vi "Ec. estados.vi"() -> ()   [LabVIEW 2020]
uses:
  <vilib>/addons/Control Design/_Model Construction/Data Typedefs.llb/CD Time Info.ctl
  <vilib>/addons/Control Design/_Model Construction/Model Creation.llb/Model Creation SubVI/cd_Create State Space Model.vi
  <vilib>/addons/Control Design/_Model Construction/Model Creation.llb/Model Creation SubVI/cd_Create Transfer Function Model.vi
  <vilib>/addons/Control Design/_Model Conversions/Model Type.llb/Model Conversion SubVI/cd_Convert Transfer Function to State-Space Model.vi
  <vilib>/addons/Control Design/_Utility/Model Viewer.llb/Model Viewer SubVI/cd_Draw State-Space Equation (SS).vi
  <vilib>/addons/Control Design/_Dynamic Analysis/Dynamic Analysis.llb/Dynamic Analysis subVI/cd_Poles (State-Space).vi
  <vilib>/addons/Control Design/_Utility/Model Viewer.llb/Model Viewer SubVI/cd_Draw Transfer Function Equation (SS).vi
  <vilib>/imath/engines/lvmath2/RunTimeEngine/Managers/WorkSpace/UID Generator.vi
  <vilib>/imath/engines/lvmath/Plug In/Control Design/BuiltInFunctions/ackermann/NIMS_CD_ackermann(A,B,poles,STR).vi
  <vilib>/imath/engines/lvmath2/RunTimeEngine/RunTimeType/NIMS_RunTimeType_From StrictType (excl LVString).vi
  <instcachedir>/0/NIMS_RunTimeType_From StrictType (excl LVString)_283B1B2000484AAA8744D21CE97EA49F.lvgen/NIMS_RunTimeType_From StrictType (excl LVString)_283B1B2000484AAA8744D21CE97EA49F_000.vi
  <vilib>/imath/engines/lvmath2/RunTimeEngine/LocalVariableDefStatement/MC_LocalVariableDefStatement_Display.vi
  <vilib>/imath/engines/lvmath2/RunTimeEngine/ArithmeticOperatorToken/NIMS_ArithmeticOperator_multmx.vi
  <instcachedir>/0/NIMS_ArithmeticOperator_multmx_177F0753FB7A49B190E35F5DD0E80316.lvgen/NIMS_ArithmeticOperator_multmx_177F0753FB7A49B190E35F5DD0E80316_004.vi
  <vilib>/imath/engines/lvmath2/RunTimeEngine/ArithmeticOperatorToken/NIMS_ArithmeticOperator_minus.vi
  <instcachedir>/0/NIMS_ArithmeticOperator_minus_822089A08BE049DB927E6BEA78E100F1.lvgen/NIMS_ArithmeticOperator_minus_822089A08BE049DB927E6BEA78E100F1_002.vi
  <vilib>/imath/engines/lvmath2/RunTimeSupport/NIMS_Get Scalar_w Error.vi
  <instcachedir>/0/NIMS_Get Scalar_w Error_5A0E401CB6154DCF81784DB8E431B6E1.lvgen/NIMS_Get Scalar_w Error_5A0E401CB6154DCF81784DB8E431B6E1_003.vi
  <vilib>/imath/engines/lvmath2/RunTimeEngine/BuiltInFunctions/ss_to_tf/NIMS_ss_to_tf(4i).vi
  <vilib>/imath/engines/lvmath2/RunTimeEngine/ErrorHandling/NIMS_Create Error From Enums.vi
  <vilib>/imath/engines/lvmath/Plug In/Control Design/BuiltInFunctions/tf/NIMS_CD_tf(num,den,Ts).vi
  <vilib>/imath/engines/lvmath/Plug In/Control Design/BuiltInFunctions/tf/NIMS_CD_tf(K,Ts).vi
  <vilib>/imath/engines/lvmath2/RunTimeEngine/VariableToken/NIMS_VariableToken_CondDefined.vi
  <instcachedir>/0/NIMS_VariableToken_CondDefined_537E119D71C74F9D9452D6FF923F1E1F.lvgen/NIMS_VariableToken_CondDefined_537E119D71C74F9D9452D6FF923F1E1F_004.vi
  <instcachedir>/0/NIMS_VariableToken_CondDefined_537E119D71C74F9D9452D6FF923F1E1F.lvgen/NIMS_VariableToken_CondDefined_537E119D71C74F9D9452D6FF923F1E1F_003.vi
  <vilib>/imath/engines/lvmath2/RunTimeSupport/NIMS_Get Any Vector_w Error - Matrix.vi
  <instcachedir>/0/NIMS_Get Any Vector_w Error - Matrix_03E716A238FA4CA1B10D931DADE97109.lvgen/NIMS_Get Any Vector_w Error - Matrix_03E716A238FA4CA1B10D931DADE97109_001.vi
  <vilib>/imath/engines/lvmath2/RunTimeEngine/ArithmeticOperatorToken/NIMS_ArithmeticOperator_power(S).vi
  <instcachedir>/0/NIMS_ArithmeticOperator_power(S)_0FB4C2FA3CD746849DC4699515FAC284.lvgen/NIMS_ArithmeticOperator_power(S)_0FB4C2FA3CD746849DC4699515FAC284_010.vi
  <vilib>/imath/engines/lvmath2/RunTimeEngine/BuiltInFunctions/abs/NIMS_abs(signed).vi
  <instcachedir>/0/NIMS_abs(signed)_C4FCB8E6058B49B797C7C8D53CA5F6EC.lvgen/NIMS_abs(signed)_C4FCB8E6058B49B797C7C8D53CA5F6EC_002.vi
  <vilib>/imathl/engines/lvmath/Functions/Error Handling/Create Error.vi
  <vilib>/imath/engines/lvmath2/RunTimeEngine/BuiltInFunctions/conv/NIMS_conv(V,V).vi
  <instcachedir>/0/NIMS_conv(V,V)_D3E194F2B5174935BB2368CEB7AAC5A9.lvgen/NIMS_conv(V,V)_D3E194F2B5174935BB2368CEB7AAC5A9_000.vi
  <vilib>/imath/engines/lvmath2/RunTimeEngine/BuiltInFunctions/roots/NIMS_roots.vi
  <instcachedir>/0/NIMS_roots_5371068BAABD481CB00E0B78F1D2DC4F.lvgen/NIMS_roots_5371068BAABD481CB00E0B78F1D2DC4F_001.vi
  <vilib>/imath/engines/lvmath/Functions/Error Handling/MergeErrorsWrapper.vi
  <vilib>/imath/engines/lvmath2/RunTimeEngine/Managers/SymbolTable/Clear UID.vi
  <vilib>/imath/engines/lvmath2/RunTimeEngine/NodeEndStatement/NIMS_NodeEndStatement_Output.vi
  <instcachedir>/0/NIMS_NodeEndStatement_Output_53EC0D466D134D7ABD903AC30B43404B.lvgen/NIMS_NodeEndStatement_Output_53EC0D466D134D7ABD903AC30B43404B_000.vi
  <instcachedir>/0/NIMS_NodeEndStatement_Output_53EC0D466D134D7ABD903AC30B43404B.lvgen/NIMS_NodeEndStatement_Output_53EC0D466D134D7ABD903AC30B43404B_010.vi
  <instcachedir>/0/NIMS_NodeEndStatement_Output_53EC0D466D134D7ABD903AC30B43404B.lvgen/NIMS_NodeEndStatement_Output_53EC0D466D134D7ABD903AC30B43404B_005.vi
  <vilib>/imath/engines/lvmath2/RunTimeEngine/ErrorHandling/NIMS_Finalize Error.vi
  <vilib>/addons/Control Design/_Utility/Model Viewer.llb/Model Viewer SubVI/cd_Draw Transfer Function Equation (TF).vi
  <vilib>/addons/Control Design/_Time Response Analysis/Time Response.llb/Time Response subVI/cd_Step Response (Transfer Function).vi
  <vilib>/addons/Control Design/_Model Construction/NI_LinSys_Model Creation.lvlib
  <vilib>/addons/Control Design/_Utility/NI_CD_Model Viewer.lvlib
  <vilib>/addons/Control Design/_State-Space Analysis/NI_CD_State-Space Analysis.lvlib
  <vilib>/addons/Control Design/_Dynamic Analysis/NI_CD_Dynamic Analysis.lvlib
  <vilib>/addons/Control Design/_Model Conversions/NI_CD_Model Type.lvlib
  <vilib>/addons/Control Design/_Time Response Analysis/NI_CD_Time Response.lvlib
  <vilib>/addons/Control Design/_Model Construction/NI_LinSys_Data Typedefs.lvlib
  <vilib>/imath/engines/lvmath2/RunTimeEngine/Managers/SymbolTable/NIMS_WorkSpace.lvlib
panel:
  out "Step Response Graph":cluster{"time":dbl[], dbl[]}[](graph)
  out "Pd":cdb[](array[numeric])
  out "FTO":picture
  in  "Observador?":bool
  in  "TF?":bool
  in  "Denominator":dbl[](array[numeric])=[1.0, 2.0, 2.0, 1.0] format="%#.5g"
  in  "Numerator":dbl[](array[numeric])=[1.0, 2.0, 1.0] format="%#.5g"
  out "FTI":picture
  in  "Polos observador":cdb[](array[numeric])=[0.0+0.0i, 0.0+0.0i, 0.0+0.0i]
  out "Ke":dbl[](array[numeric])
  out "Ki":dbl
  out "Polos Planta":cdb[](array[numeric]) format="%.3f"
  out "K":dbl[](array[numeric])
  in  "Polos  sistema":cdb[](array[numeric])=[-1.0+0.0i, -1.0+0.0i, -4.0+0.0i, -10.0+0.0i]
  out "Funcion Transferencia Planta":picture
  out "Is Observable?":bool
  out "Observability  Matrix":dbl[][](array[numeric]) format="%#.2g"
  out "Is Controllable?":bool
  out "Controllability Matrix":dbl[][](array[numeric])=[[1.0, 0.0, 6.0], [0.0, 1.0, -1.0], [0.0, 0.0, 0.0]] format="%.2f"
  out "State-Space Equation":picture
  in  "D":dbl[][](array[numeric])=[[0.0]]
  in  "C":dbl[][](array[numeric])=[[1.0, 2.0, 1.0, 0.0]]
  in  "B":dbl[][](array[numeric])=[[1.0], [0.0], [0.0], [0.0]]
  in  "A":dbl[][](array[numeric])=[[-2.0, -2.0, -1.0, 0.0], [1.0, 0.0, 0.0, 0.0], [0.0, 1.0, 0.0, 0.0], [-1.0, -2.0, -1.0, 0.0]]
  # "Funcion de Transferencia"
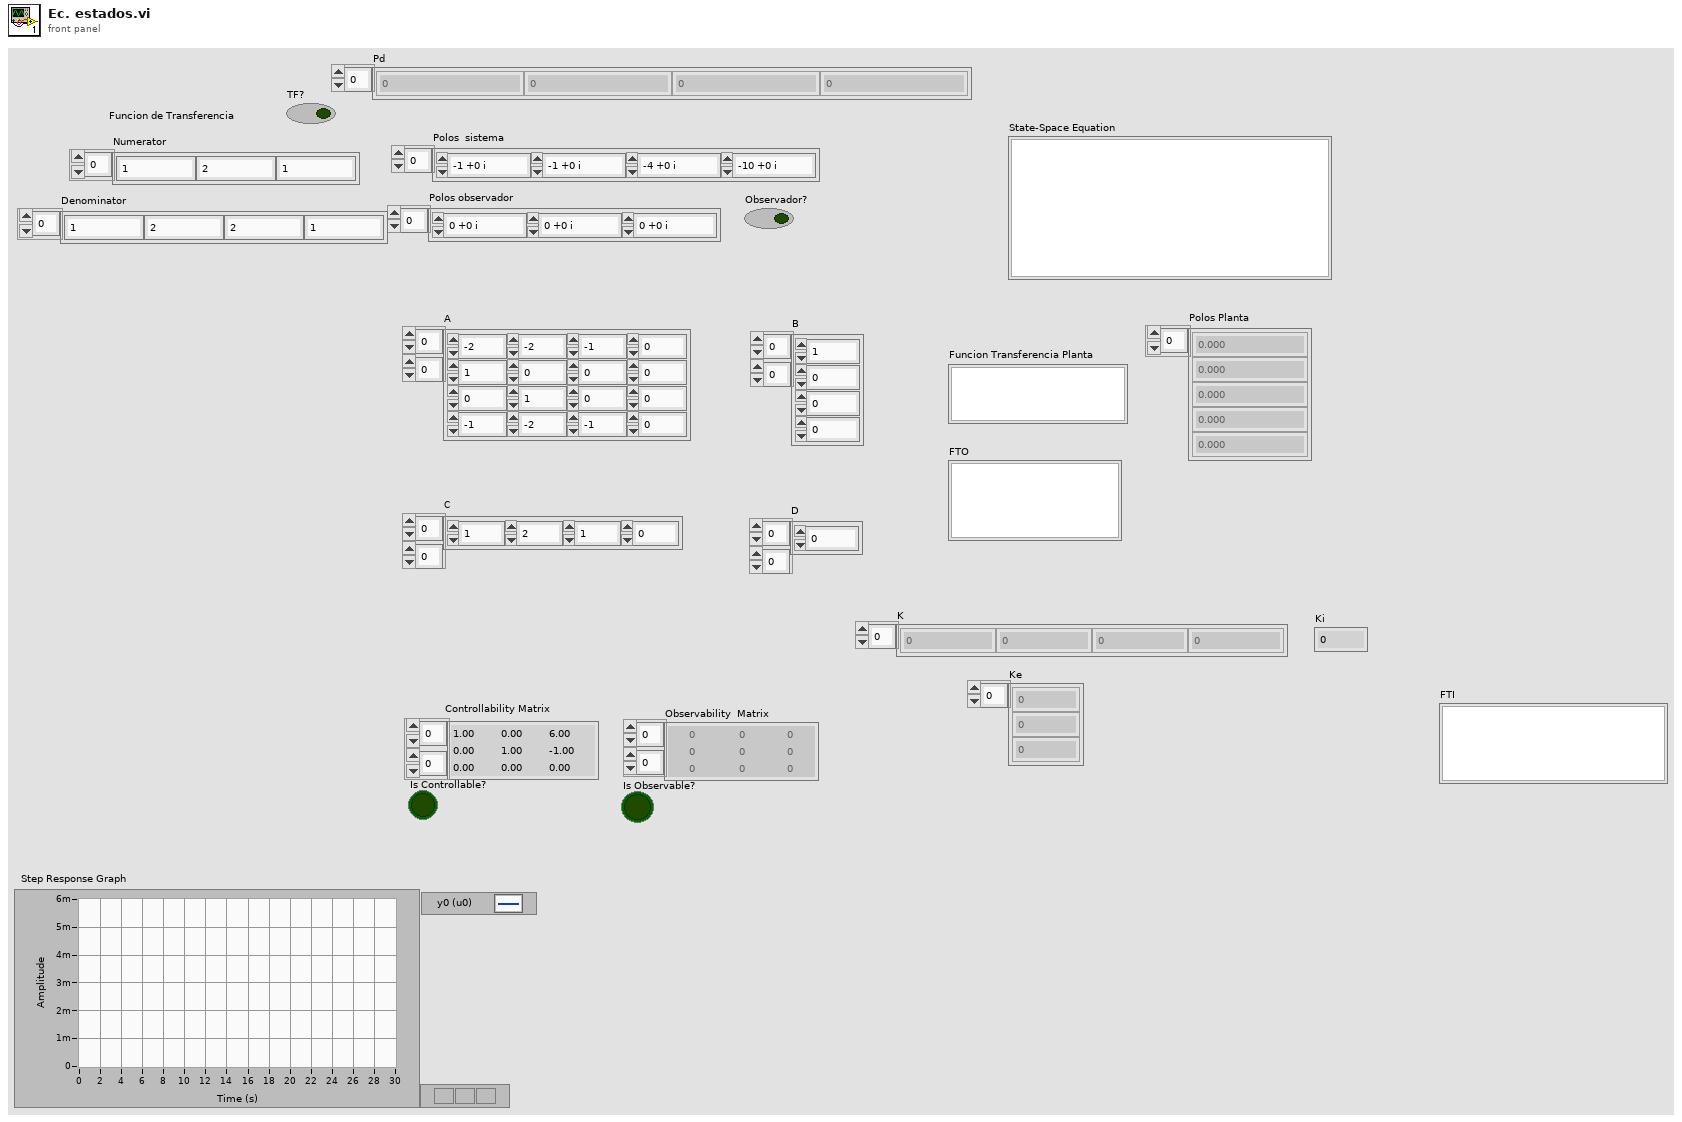
[diagram p1: front panel]
types:
  T1 = typedef "NI_LinSys_Data Typedefs.lvlib/CD Time Info.ctl" = cluster{"t0":dbl, "dt":dbl, "tf":dbl}
  T2 = typedef "NI_LinSys_Model Typedefs.lvlib/CD Transfer Function Model (MIMO).ctl" = cluster{"properties":T3, "transfer function(s)":T4[][]}
  T3 = typedef "NI_LinSys_Model Typedefs.lvlib/CD General Elements.ctl" = cluster{"Model name":string, "Input names":string[], "Output names":string[], "Input Delays":dbl[], "Output Delays":dbl[], "Sampling Time":dbl, "Notes":string}
  T4 = typedef "NI_LinSys_Model Typedefs.lvlib/CD Transfer Function Model (SISO).ctl" = cluster{"Numerator":dbl[], "Denominator":dbl[], "delay":dbl}
  T5 = typedef "NI_LinSys_Model Typedefs.lvlib/CD State Space Model (MIMO).ctl" = cluster{"properties":T3, "A":dbl[][], "B":dbl[][], "C":dbl[][], "D":dbl[][], "StateNames":string[], "Transport Delay":dbl[][]}
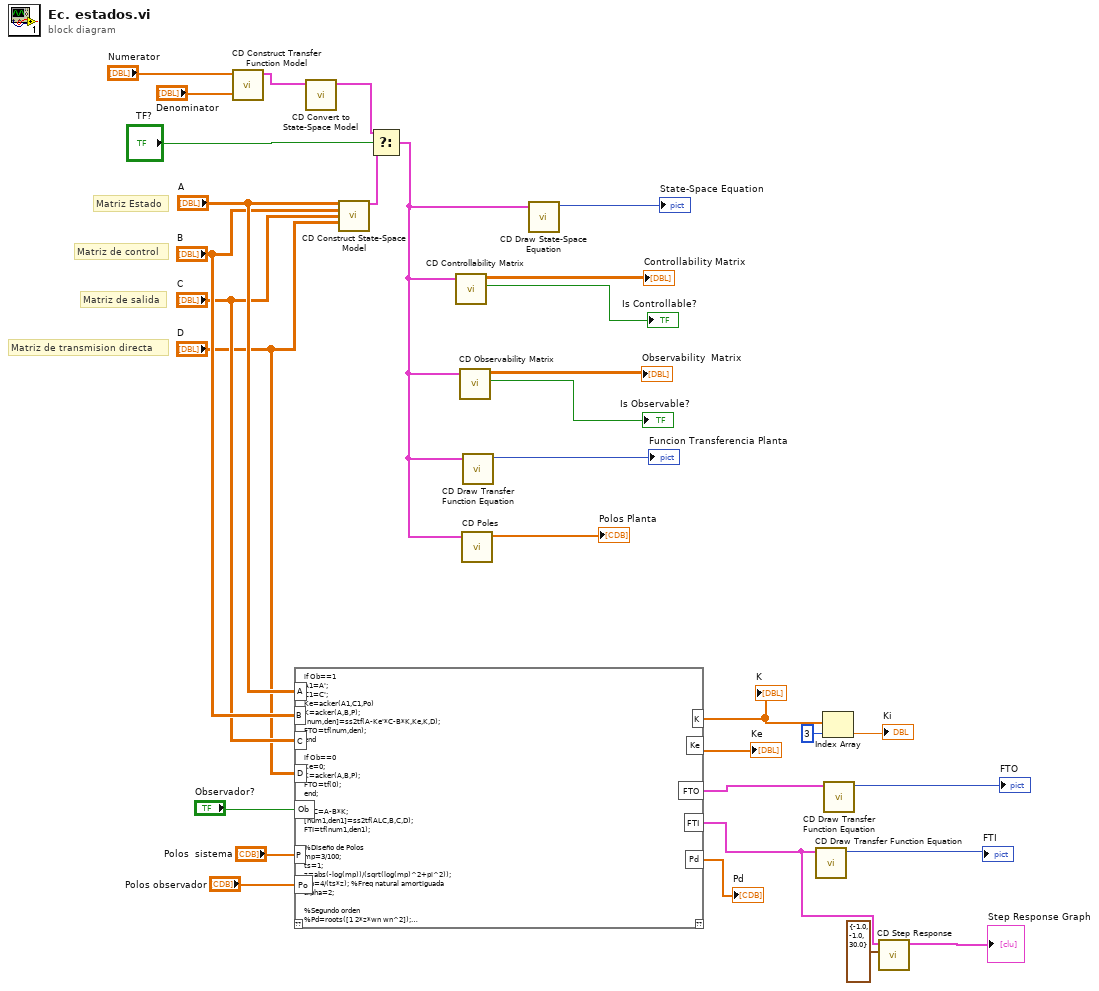
[diagram p0: block diagram]
diagram:
  # "Matriz de transmision directa"
  # "Matriz de salida"
  # "Matriz de control"
  # "Matriz Estado"
  n1 = call-poly <vilib>:"CD Construct Transfer Function Model.vi"("Denominator"="Denominator", "Numerator"="Numerator") -> ("Transfer Function Model"=w12:T2)  [unwired: 8 in, 1 out]
  n2 = mathscript code="if Ob==1 \nA1=A';\nC1=C';\nKe=acker(A1,C1,Po)\nK=acker(A,B,P);\n[num,den]=ss2tf(A-Ke'*C-B*K,Ke,K,D);\nFTO=tf(num,den);\nend\n\nif Ob==0\nKe=0;\nK=acker(A,B,P);\nFTO=tf(0);\nend;\n\nALC=A-B*K;\n[num1,den1]=ss2tf(ALC,B,C,D);\nFTI=tf(num1,den1);\n\n%Diseño de Polos\nmp=3/100;\nts=1;\nz=abs(-log(mp))/(sqrt(log(mp)^2+pi^2));\nwn=4/(ts*z); %Freq natural amortiguada\nalpha=2;\n\n%Segundo orden\n%Pd=roots([1 2*z*wn wn^2]);\n%Pd=roots(conv([1 2*z*wn wn^2, [1]]));\n\n%Tercer orden\nPd=roots(conv([1 2*z*wn wn^2], [1 alpha*wn*z]));"("A"="A", "B"="B", "P"="Polos  sistema", "C"="C", "Po"="Polos observador", "D"="D", "Ob"="Observador?") -> ("K"=w20:dbl[], "Ke"=→"Ke":dbl[], "FTI"=w2:T2, "FTO"=w7:T2, "Pd"=→"Pd":cdb[])  [unwired: 1 in, 1 out]
  "K" <- w20
  n3 = call-poly <vilib>:"CD Convert to State-Space Model.vi"("Transfer Function Model"=w12) -> ("State-Space Model"=w10:T5)  [unwired: 9 in, 1 out]
  n4 = call-poly <vilib>:"CD Construct State-Space Model.vi"("A"="A", "B"="B", "C"="C", "D"="D") -> ("State-Space Model"=w9:T5)  [unwired: 10 in, 1 out]
  n5 = Select(t=w10, s="TF?", f=w9) -> (s? t:f=w1:T5)
  n6 = call <vilib>:"CD Controllability Matrix.vi"("State-Space Model"=w1) -> ("Is Controllable?"=→"Is Controllable?":bool, "Controllability Matrix"=→"Controllability Matrix":dbl[][])  [unwired: 7 in, 2 out]
  n7 = call <vilib>:"CD Observability Matrix.vi"("State-Space Model"=w1) -> ("Is Observable?"=→"Is Observable?":bool, "Observability  Matrix"=→"Observability  Matrix":dbl[][])  [unwired: 7 in, 2 out]
  n8 = call-poly <vilib>:"CD Poles.vi"("State-Space Model"=w1) -> ("Poles"=→"Polos Planta":cdb[])  [unwired: 9 in, 1 out]
  n9 = call-poly <vilib>:"CD Draw Transfer Function Equation.vi"("State-Space Model"=w1) -> ("Equation"=→"Funcion Transferencia Planta":picture)  [unwired: 8 in, 2 out]
  n10 = call-poly <vilib>:"CD Draw State-Space Equation.vi"("State-Space Model"=w1) -> ("Equation"=→"State-Space Equation":picture)  [unwired: 8 in, 2 out]
  n11 = call-poly <vilib>:"CD Draw Transfer Function Equation.vi"("Transfer Function Model"=w2) -> ("Equation"=→"FTI":picture)  [unwired: 8 in, 2 out]
  n12 = Index Array(array=w20, index=3) -> (element=→"Ki":dbl)
  n13 = call-poly <vilib>:"CD Draw Transfer Function Equation.vi"("Transfer Function Model"=w7) -> ("Equation"=→"FTO":picture)  [unwired: 8 in, 2 out]
  n14 = call-poly <vilib>:"CD Step Response.vi"("Time Range"=T1 {"t0"=-1.0, "dt"=-1.0, "tf"=30.0}, "Transfer Function Model"=w2) -> ("Step Response Graph"=→"Step Response Graph":cluster{"time":dbl[], dbl[]}[])  [unwired: 7 in, 2 out]
